vi "wSetup.vi"(0 "Socket_000 in":refnum<class "TCPAlerts.lvclass">, 5 "IP Address":string, 7 "Port":u16, 11 "error in (no error)":errorcluster) -> (4 "Socket_000 out":refnum<class "TCPAlerts.lvclass">, 15 "error out":errorcluster)   [LabVIEW 2011, in "TCPAlerts.lvclass"]
uses:
  TCPAlerts.lvclass
  TCPAlerts.lvclass/TCPAlerts.ctl
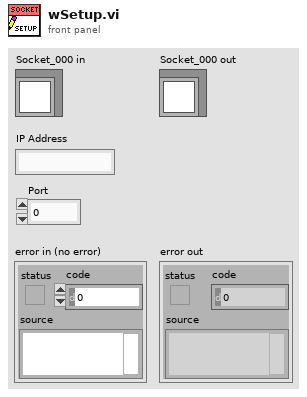
[diagram p1: front panel]
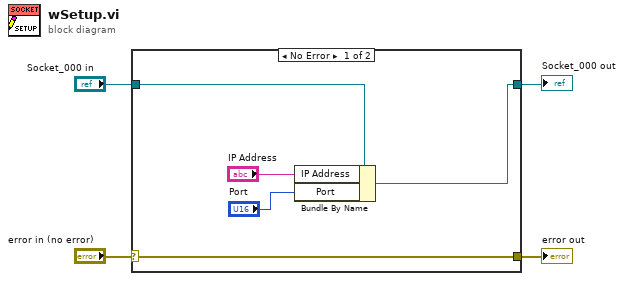
[diagram p0: block diagram]
diagram:
  n1 = case shown="No Error" "error in (no error)" {
    selector: "error in (no error)" -> [w9 w10]
    tunnel: [w9 w10] -> w1
    tunnel: [w7 w11] -> w4
    tunnel: "Socket_000 in" -> [w8 w11]
    frame No Error {
      n2 = Bundle By Name(cluster=w8, "IP Address"="IP Address", "Port"="Port") -> (w7:refnum<class "TCPAlerts.lvclass">)
    }
    frame Error {
    }
  }
  "error out" <- w1
  "Socket_000 out" <- w4
